vi "Alarm interface.vi"(8 "错误输入（无错误）":errorcluster, 9 "code":i32, 10 "模块名称":string) -> (0 "错误输出":errorcluster)   [LabVIEW 2016, in "质控单元V1.lvlib"]
panel:
  in  "簇":T1
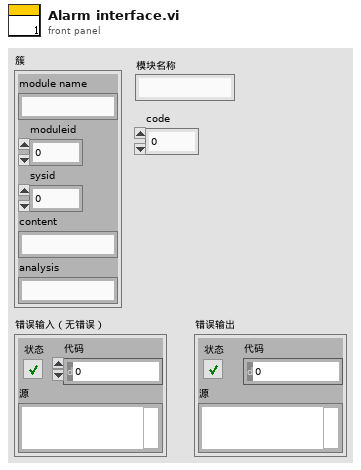
[diagram p1: front panel]
types:
  T1 = cluster{"module name":string, "moduleid":i32, "sysid":i32, "content":string, "analysis":string}
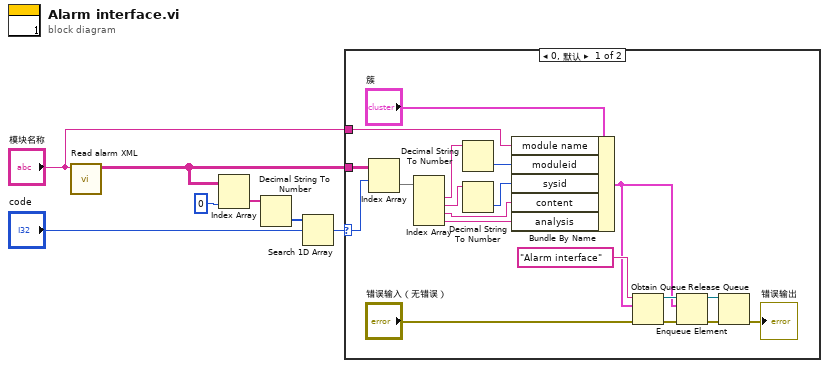
[diagram p0: block diagram]
diagram:
  n1 = call "Read alarm XML.vi"("模块名称"="模块名称") -> ("报警输出"=w1:string[][])  [unwired: 10 in]
  n2 = Index Array(array=w1, index (col)=0 ("禁用的索引 (列)")) -> (element=w6:string[])  [unwired: 1 in]
  n3 = Decimal String To Number(string=w6) -> (number=w5:i32[])  [unwired: 2 in, 1 out]
  n4 = Search 1D Array(1D array=w5, element="code") -> (index of element=w3:i32)  [unwired: 1 in]
  n5 = case shown="0, 默认" w3 {
    selector: w3 -> [w8 _]
    tunnel: "模块名称" -> [w10 _]
    tunnel: w1 -> [w9 _]
    frame 0, Default {
      n6 = Index Array(array=w9, index (row)=w8) -> (element=w26:string[])  [unwired: 1 in]
      n7 = Index Array(array=w26) -> (element #1=w25:string, element #2=w24:string, element #3=w21:string, element #4=w20:string)  [unwired: 4 in]
      n8 = Decimal String To Number(string=w25) -> (number=w23:i32)  [unwired: 2 in, 1 out]
      n9 = Decimal String To Number(string=w24) -> (number=w22:i32)  [unwired: 2 in, 1 out]
      n10 = Bundle By Name(cluster="簇", "module name"=w10, "moduleid"=w23, "sysid"=w22, "content"=w21, "analysis"=w20) -> (w11:T1)
      n11 = Obtain Queue(name (unnamed)="Alarm interface" ("名称（未命名）"), element data type=w11, error in (no error)="错误输入（无错误）") -> (queue out=w15:refnum<queue>, error out=w14:errorcluster)  [unwired: 2 in, 1 out]
      n12 = Enqueue Element(queue=w15, element=w11, error in (no error)=w14) -> (queue out=w13:refnum<queue>, error out=w12:errorcluster)  [unwired: 1 in, 1 out]
      n13 = Release Queue(queue=w13, error in (no error)=w12) -> (error out=→"错误输出":errorcluster)  [unwired: 1 in, 2 out]
    }
    frame -1 {
    }
  }
